vi "215.Syringe (SubVI).vi"(7 "Source":string(combo), 8 "error in (no error)":errorcluster, 9 "Syringe Cycle (ms)":u16=1000, 10 "Flush Volume":i32=100, 11 "VISA Refnum in":refnum<visa-resource-name>) -> (0 "error out":errorcluster, 2 "String":string, 3 "VISA Refnum out":refnum<visa-resource-name>)   [LabVIEW 2020]
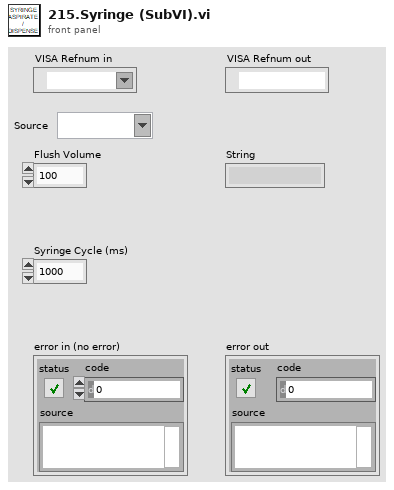
[diagram p1: front panel]
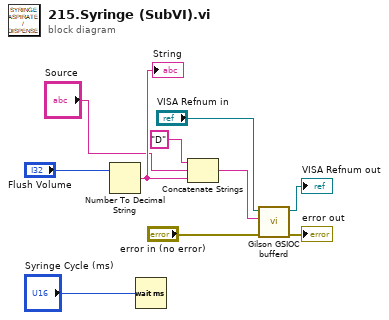
[diagram p0: block diagram]
diagram:
  n1 = Number To Decimal String(number="Flush Volume") -> (decimal integer string=w10:string)  [unwired: 1 in]
  "String" <- w10
  n2 = Wait (ms)(milliseconds to wait="Syringe Cycle (ms)") -> ()  [unwired: 1 out]
  n3 = Concatenate Strings("D" ("string"), "Source", w10) -> (w3:string)
  n4 = call <instrlib>:"Gilson GSIOC bufferd.vi"("error in (no error)"="error in (no error)", "Bufferd command"=w3, "VISA resource name"="VISA Refnum in") -> ("error out"=→"error out":errorcluster, "VISA resource name out"=→"VISA Refnum out":refnum<visa-resource-name>)  [unwired: 6 in, 1 out]
